vi "provide_note_book_info.vi"(8 "error in (no error)":errorcluster, 10 "notebook string in":string, 11 "GenericPlugin in":refnum<class "StimulatorDL090824Gate.lvclass">) -> (0 "error out":errorcluster, 2 "notebook string out":string, 3 "GenericPlugin out":refnum<class "StimulatorDL090824Gate.lvclass">)   [LabVIEW 2010, in "StimulatorDL090824Gate.lvclass"]
uses:
  StimulatorDL090824Gate.lvclass
  StimulatorDL090824Gate.lvclass/StimulatorDL090824Gate.ctl
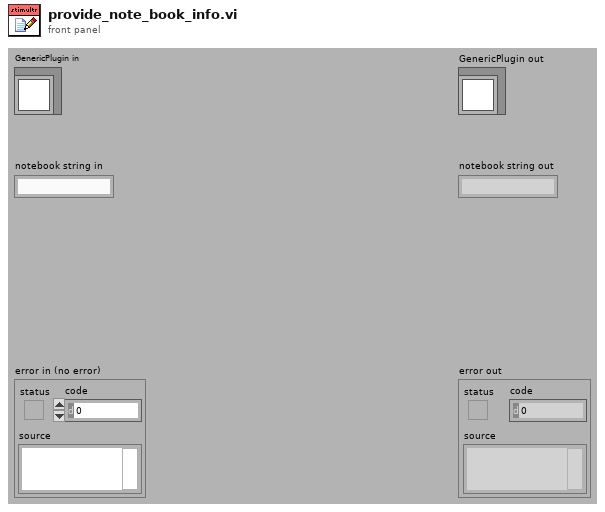
[diagram p1: front panel]
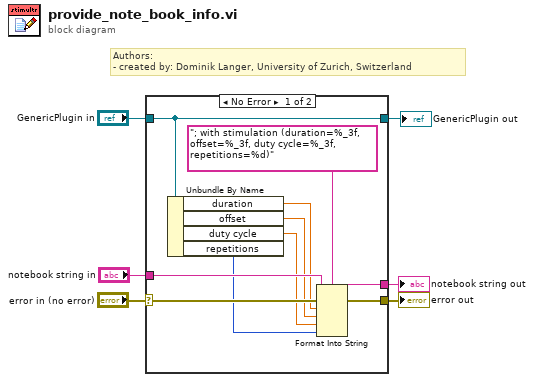
[diagram p0: block diagram]
diagram:
  # "Authors: \n- created by: Dominik Langer, University of Zurich, Switzerland"
  n1 = case shown="No Error" "error in (no error)" {
    selector: "error in (no error)" -> [w14 w19]
    tunnel: "GenericPlugin in" -> [w13 w18]
    tunnel: [w16 w19] -> w4
    tunnel: "notebook string in" -> [w15 w17]
    tunnel: [w13 w18] -> w2
    tunnel: [w7 w17] -> w1
    frame No Error {
      n2 = Unbundle By Name(w13) -> ("duration"=w12:dbl[unit], "offset"=w11:dbl[unit], "duty cycle"=w10:dbl[unit], "repetitions"=w9:i32)
      n3 = Format Into String(format string="; with stimulation (duration=%_3f, offset=%_3f, duty cycle=%_3f, repetitions=%d)", initial string=w15, error in=w14, w12, w11, w10, w9) -> (resulting string=w7:string, error out=w16:errorcluster)
    }
    frame Error {
    }
  }
  "error out" <- w4
  "GenericPlugin out" <- w2
  "notebook string out" <- w1
